vi "Initialize.vi"(8 "error in (no error)":errorcluster, 10 "Serial Port":string, 11 "Serial Device in":refnum<class "Simulated Serial Device.lvclass">) -> (0 "error out":errorcluster, 3 "Serial Device out":refnum<class "Simulated Serial Device.lvclass">)   [LabVIEW 2017, in "Simulated Serial Device.lvclass"]
uses:
  Simulated Serial Device.lvclass
  C:/LGP5/Resources/Unit-Testing/Serial Project/Libraries/Serial Device_class/Serial Device.lvclass
  Serial Device_class/Serial Device.lvclass/Serial Device.ctl
  Serial Device_class/Set Serial Port.vi
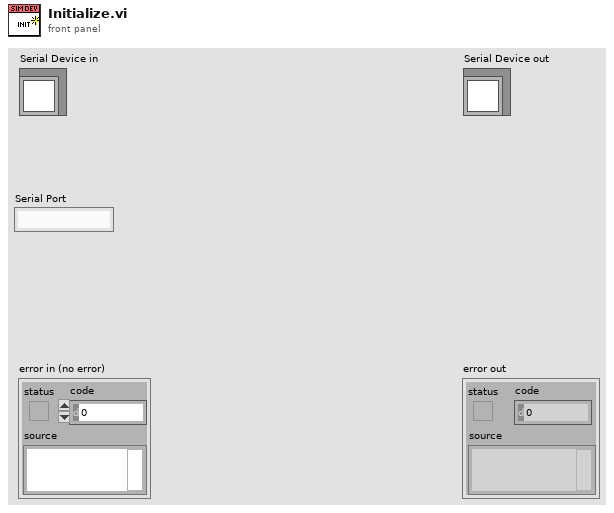
[diagram p1: front panel]
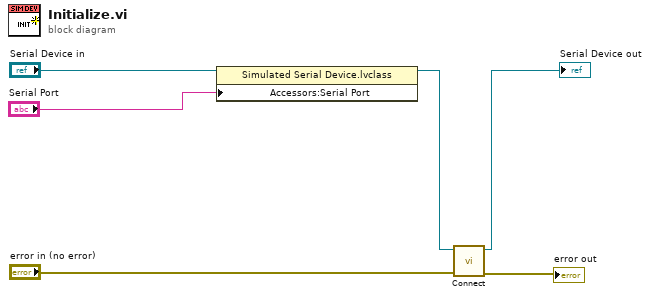
[diagram p0: block diagram]
diagram:
  n1 = property class="Simulated Serial Device.lvclass"(reference="Serial Device in", "Accessors:Serial Port"="Serial Port") -> (reference out=w2:refnum<class "Simulated Serial Device.lvclass">)  [unwired: 1 in, 1 out]
  n2 = call-dynamic "Connect.vi"("error in (no error)"="error in (no error)", "Simulated Serial Device in"=w2) -> ("error out"=→"error out":errorcluster, "Simulated Serial Device out"=→"Serial Device out":refnum<class "Simulated Serial Device.lvclass">)  [unwired: 8 in]
